vi "conv EOL.vi"(10 "standard output in":string) -> (2 "result string":string)   [LabVIEW 2020, in "Approval Tests.lvlib"]
uses:
  Approval Tests.lvlib
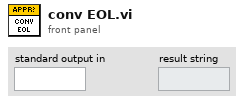
[diagram p1: front panel]
types:
  T1 = enum16{"Native", "Native Command Line", "UNIX", "Macintosh", "DOS"}
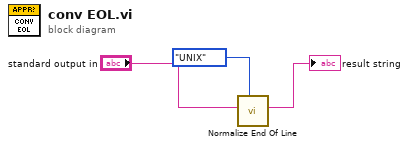
[diagram p0: block diagram]
diagram:
  n1 = call <vilib>:"Normalize End Of Line.vi"("end of line (Native)"=T1."UNIX", "string in"="standard output in") -> ("string out"=→"result string":string)  [unwired: 6 in]
